vi "IsEventCtrlValid.vi"(8 "error in (no error)":errorcluster, 11 "Control in":refnum<vi>) -> (0 "error out":errorcluster, 2 "Boolean":bool)   [LabVIEW 2016, in "LV Object Event Registration Node.xnode"]
uses:
  LV Object Event Registration Node.xnode
  <vilib>/Utility/Data Type/Type Definitions/Refnum Type.ctl
  <vilib>/Utility/Data Type/NI_Data Type.lvlib
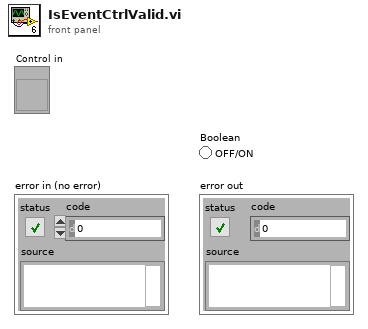
[diagram p1: front panel]
types:
  T1 = typedef "NI_Data Type.lvlib/Refnum Type.ctl" = enum16{"NotARefnum", "UnknownRefnum", "Generic", "Datalog", "ByteStream", "Device", "Occurence", "TCPNetConnection", "Auto", "Menu", "Imaq", "Hardware", "DataSocket", "Visa", "IVI", "UDPNetConnection", "Notifier", "Queue", "Irda", "EventReg", "DotNet", "UserEvent", "Callback", "UNUSED_EMPTY_POSITION", "BlueToothNetConnection", "LVObjApp", "LVObjVI", "LVObjUnknown", "GenericClass", "UserDefinedRefnumTag", "DataValue", "RT FIFO", "TDMS File"}
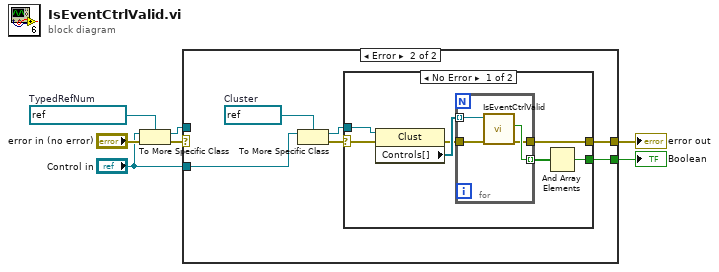
[diagram p0: block diagram]
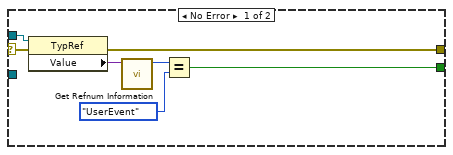
[diagram p2: hidden frame]
diagram:
  w2 = refnum<vi> refnum  # TypedRefNum
  n1 = To More Specific Class(target class=w2, reference="Control in", error in="error in (no error)") -> (specific class reference=w4:refnum<vi>, error out=w3:errorcluster)
  n2 = case shown="Error" w3 {
    selector: w3 -> [w9 _]
    tunnel: w4 -> [w11 _]
    tunnel: [w10 w16] -> w5
    tunnel: [w8 w15] -> w7
    tunnel: "Control in" -> [_ w20]
    frame No Error {
      n3 = property class="TypRef"(reference=w11, error in=w9) -> (error out=w8:errorcluster, "Value"=w12:variant)  [unwired: 1 out]
      n4 = call <vilib>:"Get Refnum Information.vi"("Variant"=w12) -> ("Reference Type"=w13:T1)  [unwired: 7 in, 3 out]
      n5 = Equal?(x=w13, y=Refnum_Type."UserEvent") -> (x = y?=w10:bool)
    }
    frame Error {
      w19 = refnum<vi> refnum  # Cluster
      n6 = To More Specific Class(target class=w19, reference=w20) -> (specific class reference=w17:refnum<vi>, error out=w18:errorcluster)  [unwired: 1 in]
      n7 = case shown="No Error" w18 {
        selector: w18 -> [w23 _]
        tunnel: w17 -> [w27 _]
        tunnel: [w24 _] -> w16
        tunnel: [w21 _] -> w15
        frame No Error {
          n8 = property class="Clust"(reference=w27, error in=w23) -> (error out=w22:errorcluster, "Controls[]"=w26:refnum<vi>[])  [unwired: 1 out]
          n9 = for {
            tunnel: w26 -> [w31] mode=indexing
            tunnel: [w30] -> w25 mode=indexing
            tunnel: w22 -> [w29]
            tunnel: [w28] -> w21
            n10 = call "IsEventCtrlValid.vi"("error in (no error)"=w29, "Control in"=w31) -> ("error out"=w28:errorcluster, "Boolean"=w30:bool)  [unwired: 8 in]
          }
          n11 = And Array Elements(Boolean array=w25) -> (logical AND=w24:bool)
        }
        frame Error {
        }
      }
    }
  }
  "error out" <- w7
  "Boolean" <- w5
